vi "Draw Textured Triangle.vi"(9 "Texture":T5, 10 "Triangle":T1={"Vertex 1"={"Position"={"x"=0.0, "y"=0.0, "z"=0.0}, "UV"={"u"=0.0, "v"=0.0}, "Colour"=12517256}, "Vertex 2"={"Position"={"x"=0.0, "y"=0.0, "z"=0.0}, "UV"={"u"=0.0, "v"=0.0}, "Colour"=12517256}, "Vertex 3"={"Position"={"x"=0.0, "y"=0.0, "z"=0.0}, "UV"={"u"=0.0, "v"=0.0}, "Colour"=12517256}, "Colour"=0} {"Vertex 3"."UV"."v" min=0 max=1 step=0.1; "Vertex 3"."UV"."u" min=0 max=1 step=0.1; "Vertex 2"."UV"."v" min=0 max=1 step=0.1; "Vertex 2"."UV"."u" min=0 max=1 step=0.1; "Vertex 1"."UV"."v" min=0 max=1 step=0.1; "Vertex 1"."UV"."u" min=0 max=1 step=0.1}, 11 "Pixel Data in":u32[][](array[numeric])) -> (3 "Pixel Data out":u32[][](array[numeric]))   [LabVIEW 2020]
uses:
  Raster (FPGA).lvlib
  Libraries/Utility/Utility.lvlib
  UV.ctl
  <vilib>/Utility/miscctls.llb/LVPointTypeDef.ctl
  Rectangle Dimensions.ctl
  Texture.ctl
  Vector 3D.ctl
  Vertex.ctl
  Triangle.ctl
panel:
  out "new picture":picture
  in  "Zoom Factor":sgl=5.0
  in  "Origin":T7={"Horizontal"=0, "Vertical"=426}
  # "(0,1)"
  # "(1,1)"
  # "(0,0)"
  # "(1,0)"
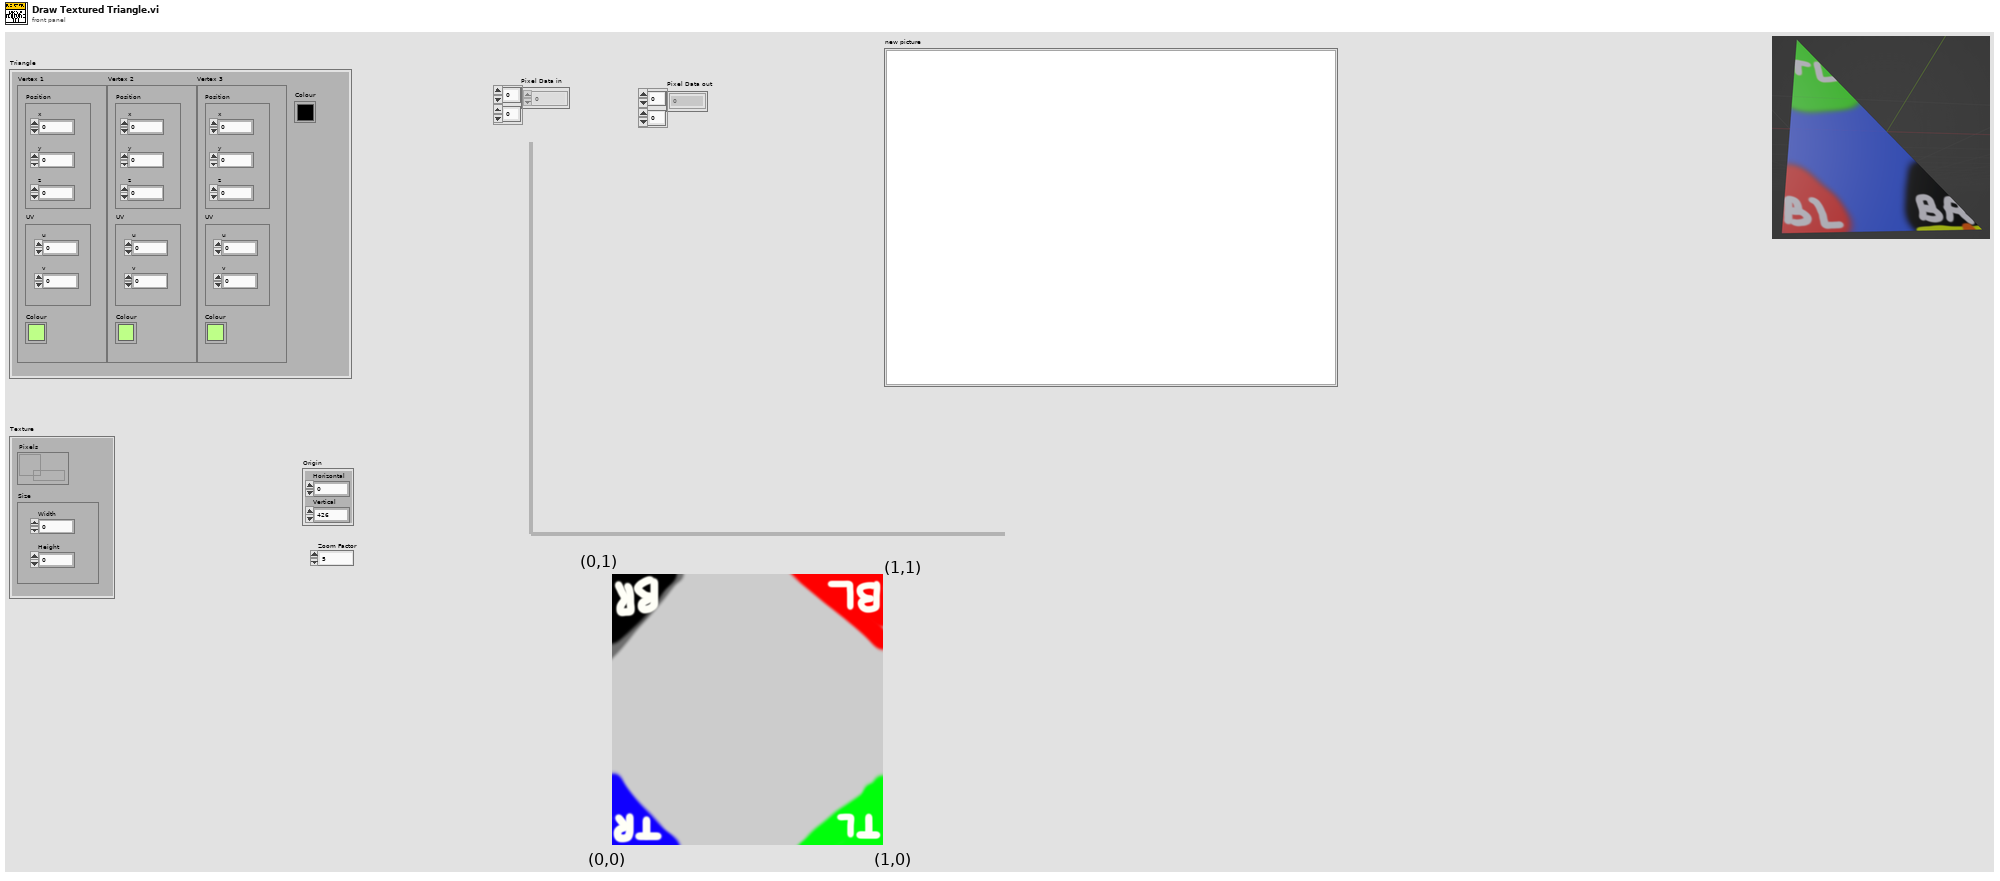
[diagram p1: front panel]
types:
  T1 = typedef "Raster (FPGA).lvlib/Triangle.ctl" = cluster{"Vertex 1":T2, "Vertex 2":T2, "Vertex 3":T2, "Colour":u32}
  T2 = typedef "Raster (FPGA).lvlib/Vertex.ctl" = cluster{"Position":T3, "UV":T4, "Colour":u32}
  T3 = typedef "Raster (FPGA).lvlib/Vector 3D.ctl" = cluster{"x":sgl, "y":sgl, "z":sgl}
  T4 = typedef "Raster (FPGA).lvlib/UV.ctl" = cluster{"u":sgl, "v":sgl}
  T5 = typedef "Raster (FPGA).lvlib/Texture.ctl" = cluster{"Pixels":refnum<data-value>, "Size":T6}
  T6 = typedef "Raster (FPGA).lvlib/Rectangle Dimensions.ctl" = cluster{"Width":u32, "Height":u32}
  T7 = typedef "LVPointTypeDef.ctl" = cluster{"Horizontal":i16, "Vertical":i16}
  T8 = typedef "3D (FPGA).lvlib/Triangle (Sorted).ctl" = cluster{"Top Vertex":T2, "Mid Vertex":T2, "Bottom Vertex":T2, "Colour":u32}
  T9 = typedef "Raster (FPGA).lvlib/Reciprocals.ctl" = cluster{"Bottom --> Top":sgl, "Bottom --> Middle":sgl, "Middle --> Top":sgl}
  T10 = typedef "Raster (FPGA).lvlib/Texel Step Deltas (BMT).ctl" = cluster{"Bottom To Top":T11, "Bottom To Middle":T11, "Middle To Top":T11}
  T11 = typedef "Raster (FPGA).lvlib/Point 2D (SGL).ctl" = cluster{"x":sgl, "y":sgl}
  T12 = typedef "Raster (FPGA).lvlib/Texel Step Deltas.ctl" = cluster{"Texel Start":T11, "Texel End":T11}
  T13 = typedef "Raster (FPGA).lvlib/Current Row.ctl" = cluster{"Start Column":sgl, "End Column":sgl}
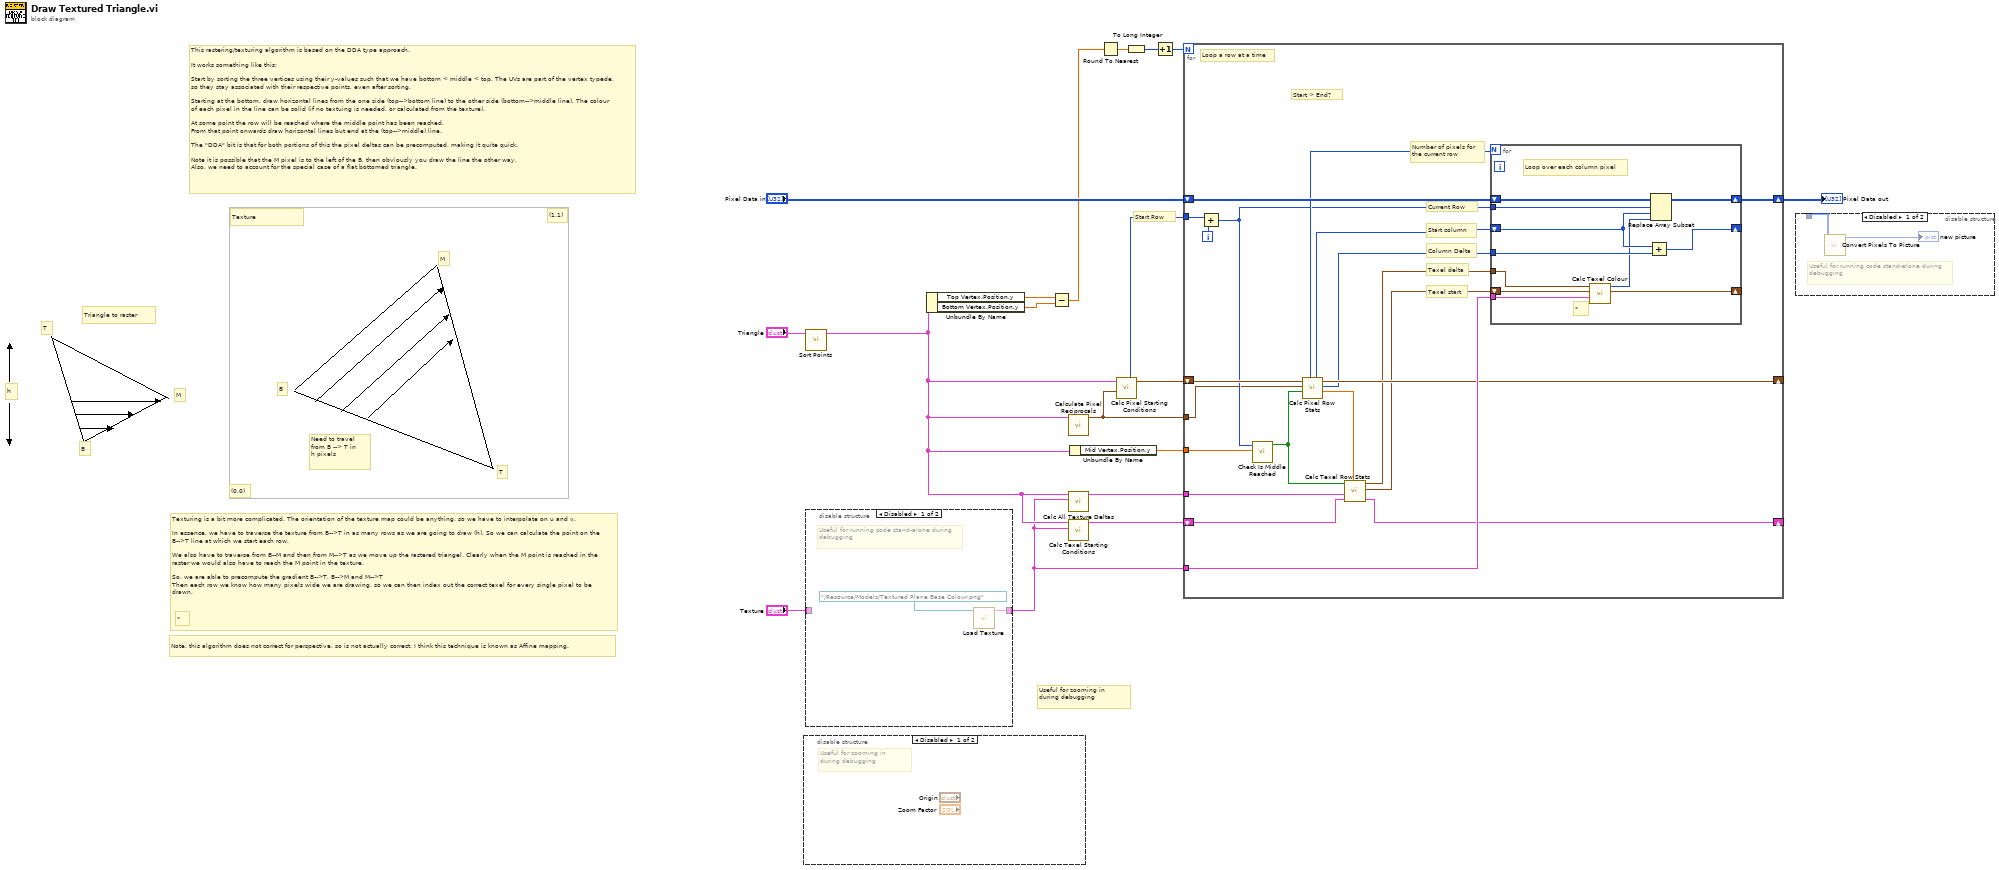
[diagram p0: block diagram]
diagram:
  # "Note, this algorithm does not correct for perspective, so is not actually correct. I think this technique is known as Affine mapping."
  # "*"
  # "Texturing is a bit more complicated. The orientation of the texture map could be anything, so we have to interpolate on u and v.\n\nIn essence, we have to traverse the texture from B-->T in as many rows as we are going to draw (h). So we can calculate the point on the B-->T line at which we start each row.\n\nWe also have to traverse from B--M and then from M-->T as we move up the rastered triangel. Clearly when the M point is reached in the raster we would also have to reach the M point in the texture.\n\nSo, we are able to precompute the gradient B-->T, B-->M and M-->T\nThen each row we know how many pixels wide we are drawing, so we can then index out the correct texel for every single pixel to be drawn."
  # "(0,0)"
  # "(1,1)"
  # "h"
  # "Texture"
  # "Triangle to raster"
  # "M"
  # "T"
  # "B"
  # "Need to travel from B --> T in \nh pixels"
  # "T"
  # "M"
  # "B"
  # "This rastering/texturing algorithm is based on the DDA type approach.\n\nIt works something like this:\n\nStart by sorting the three vertices using their y-values such that we have bottom < middle < top. The UVs are part of the vertex typede, so they stay associated with their respective points, even after sorting.\n\nStarting at the bottom, draw horizontal lines from the one side (top-->bottom line) to the other side (bottom-->middle line). The colour of each pixel in the line can be solid (if no textuing is needed, or calculated from the texture).\n\nAt some point the row will be reached where the middle point has been reached.\nFrom that point onwards draw horizontal lines but end at the (top-->middle) line.\n\nThe \"DDA\" bit is that for both portions of this the pixel deltas can be precomputed, making it quite quick.\n\nNote it is possible that the M pixel is to the left of the B, then obviously you draw the line the other way.\nAlso, we need to account for the special case of a flat bottomed triangle."
  # "Useful for zooming in during debugging"
  # "Start Row"
  n1 = disable-structure shown="Disabled" {
    frame Disabled {
      # "Useful for zooming in during debugging"
    }
    frame Enabled {
    }
  }
  n2 = call "Sort Points.vi"("Triangle"="Triangle") -> ("Sorted Triangle"=w5:T8)  [unwired: 10 in]
  n3 = disable-structure shown="Disabled" {
    disable-tunnel: "Texture" -> [_ w23]
    disable-tunnel: [w22 w23] -> w4
    frame Disabled {
      # "Useful for running code stand-alone during debugging"
      n4 = call "Load Texture.vi"("Texture Name"=path "../Resource/Models/Textured Plane Base Colour.png" ("name or relative path")) -> ("Texture"=w22:T5)  [unwired: 10 in]
    }
    frame Enabled {
    }
  }
  n5 = Unbundle By Name(w5) -> ("Top Vertex.Position.y"=w9:sgl, "Bottom Vertex.Position.y"=w8:sgl)
  n6 = Subtract(x=w9, y=w8) -> (x-y=w2:sgl)
  n7 = call "Calculate Pixel Reciprocals.vi"("Sorted Triangle"=w5) -> ("Columns Pixels Per Row"=w16:T9)  [unwired: 10 in]
  n8 = call "Calc All Texture Deltas.vi"("Texture"=w4, "Sorted Triangle"=w5) -> ("Texels Step Deltas"=w11:T10)  [unwired: 9 in]
  n9 = call "Calc Texel Starting Conditions.vi"("Texture"=w4, "Sorted Triangle"=w5) -> ("Step Deltas (Texels Per Step)"=w12:T12)  [unwired: 9 in]
  n10 = Unbundle By Name(w5) -> ("Mid Vertex.Position.y"=w7:sgl)
  n11 = Round To Nearest(number=w2) -> (nearest integer value=w3:sgl)
  n12 = call "Calc Pixel Starting Conditions.vi"("Reciprocals"=w16, "Sorted Vertices (V1 is top)"=w5) -> ("Start Row Columns"=w17:T13, "Start Row"=w18:i32)  [unwired: 8 in]
  n13 = To Long Integer(number=w3) -> (32bit integer=w1:i32)
  n14 = Increment(x=w1) -> (x+1=w14:i32)
  n15 = for {
    N: w14 -> [_]
    shift-right: [w42] -> w13
    shift-left: "Pixel Data in" -> [w43]
    tunnel: w4 -> [w41]
    tunnel: w18 -> [w40]
    shift-right: [w36] -> _
    shift-left: w17 -> [w38]
    tunnel: w7 -> [w33]
    tunnel: w16 -> [w32]
    shift-right: [w29] -> _
    shift-left: w12 -> [w28]
    tunnel: w11 -> [w31]
    i -> [w39]
    # "Column Delta"
    # "Start > End?"
    # "Current Row"
    # "Texel delta"
    # "Texel start"
    # "Start column"
    # "Loop a row at a time"
    # "Number of pixels for the current row"
    n16 = Add(x=w40, y=w39) -> (x+y=w34:i32)
    n17 = call "Check Is Middle Reached.vi"("Middle y"=w33, "Current Row"=w34) -> ("Reached Middle"=w26:bool)  [unwired: 9 in]
    n18 = call "Calc Pixel Row Stats.vi"("Reached Middle"=w26, "Reciprocals"=w32, "Current Row"=w38) -> ("Row width (pixels)"=w30:sgl, "Column Delta"=w25:i32, "Next Row"=w36:T13, "Start Col"=w24:i32, "Number Of Cols This Row"=w37:i32)  [unwired: 4 in]
    n19 = call "Calc Texel Row Stats.vi"("Row width (pixels)"=w30, "Step Deltas (Texels Per Step) in"=w28, "Texels Step Deltas"=w31, "Reached Middle"=w26) -> ("Step Deltas (Texels Per Step) out"=w29:T12, "Texel Start"=w35:T11, "Texel Delta Per Pixel"=w27:T11)  [unwired: 5 in]
    n20 = for {
      N: w37 -> [_]
      shift-right: [w47] -> w42
      shift-left: w43 -> [w48]
      tunnel: w41 -> [w51]
      tunnel: w34 -> [w46]
      tunnel: w27 -> [w53]
      shift-right: [w54] -> _
      shift-left: w35 -> [w52]
      shift-right: [w50] -> _
      shift-left: w24 -> [w45]
      tunnel: w25 -> [w49]
      # "*"
      # "Loop over each column pixel"
      # "cols"
      n21 = call "Calc Texel Colour.vi"("Texture"=w51, "Texel Start"=w52, "Texel Delta Per Pixel in"=w53) -> ("Texel Delta Per Pixel out"=w54:T11, "Colour"=w44:u32)  [unwired: 7 in]
      n22 = Add(x=w45, y=w49) -> (x+y=w50:i32)
      n23 = Replace Array Subset(array=w48, new element=w44, index (row)=w46, index (col)=w45) -> (w47:u32[][])
    }
  }
  "Pixel Data out" <- w13
  n24 = disable-structure shown="Disabled" {
    disable-tunnel: _ -> [w55 _]
    frame Disabled {
      # "Useful for running code stand-alone during debugging"
      n25 = call "Convert Pixels To Picture.vi"("Pixel Data in"=w55) -> ("2D Picture"=→"new picture":picture)  [unwired: 9 in, 1 out]
    }
    frame Enabled {
    }
  }
